vi "WriteJSON.vi"(2 "error in (no error)":errorcluster, 3 "JSONEventInfo":variant) -> (0 "error out":errorcluster, 1 "Boolean":bool)   [LabVIEW 2018]
uses:
  <vilib>/LVH/i3 JSON/JSON Parsing/Get Object Parameter Files/Get Object Parameter - String.vi
  Global Variables.vi
  <vilib>/LVH/i3 JSON/JSON Generation/Create Value Files/Create Value - Object.vi
  <vilib>/LVH/i3 JSON/JSON Generation/Add Object Parameter Files/Add Object Parameter - Object.vi
  <vilib>/LVH/i3 JSON/JSON Generation/Add Object Parameter Files/Add Object Parameter - String.vi
  <vilib>/LVH/i3 JSON/JSON Generation/Append to Array Files/Append to Array - Object.vi
  <vilib>/LVH/i3 JSON/i3-json.lvlib
panel:
  out "JSONpath":path
  in  "String 2":string
  out "concatenated string":string
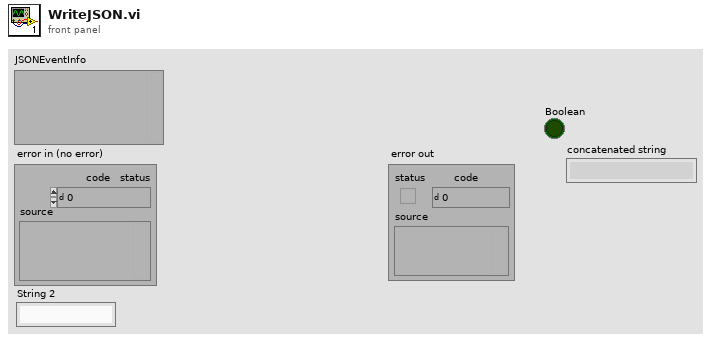
[diagram p1: front panel]
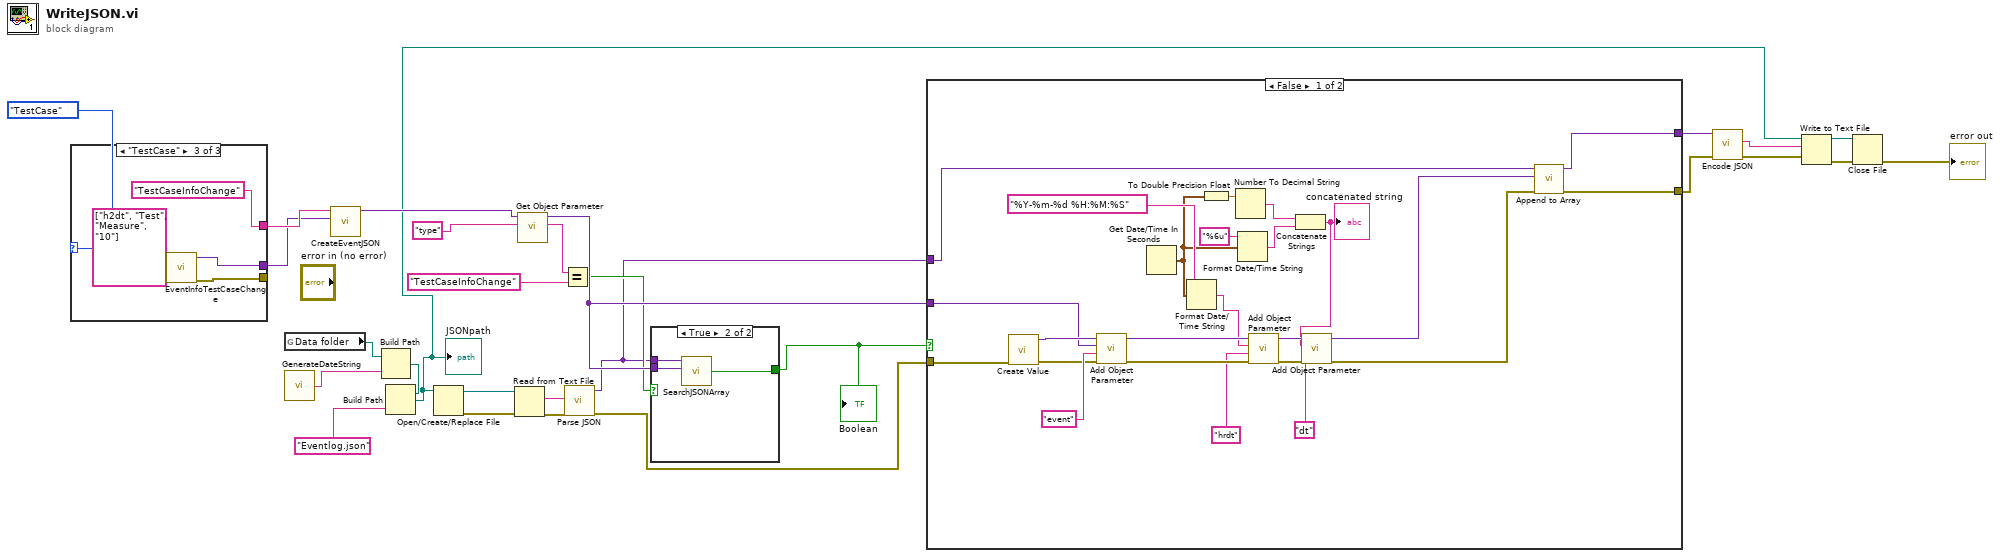
[diagram p0: block diagram]
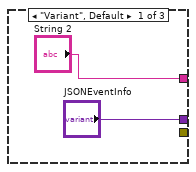
[diagram p3: hidden frame]
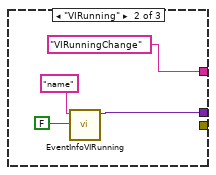
[diagram p4: hidden frame]
diagram:
  n1 = case shown="\"TestCase\"" enum16{"Variant", "TestCase", "VIRunning"}."TestCase" {
    tunnel: ["JSONEventInfo" w34 w38] -> w12
    tunnel: [_ _ w36] -> _
    tunnel: ["String 2" "VIRunningChange" "TestCaseInfoChange"] -> w13
    frame "Variant", Default {
    }
    frame "VIRunning" {
      n2 = call "EventInfoVIRunning.vi"("OnOff"=FALSE, "name"="name") -> ("eventinfoJSON"=w34:variant)  [unwired: 8 in, 1 out]
    }
    frame "TestCase" {
      n3 = call "EventInfoTestCaseChange.vi"("TestCaseInfo"=string[] ["h2dt", "Test", "Measure", "10"]) -> ("error out"=w36:errorcluster, "JSON Tree out (JSON Object)"=w38:variant)  [unwired: 9 in]
    }
  }
  n4 = global read "Global Variables.vi" "Data folder"() -> (w27:path)
  n5 = call "GenerateDateString.vi"() -> ("String"=w28:string)
  n6 = call "CreateEventJSON.vi"("eventinfo"=w12, "type"=w13) -> ("eventJSON"=w14:variant)  [unwired: 8 in, 1 out]
  n7 = Build Path(base path=w27, name or relative path=w28) -> (appended path=w26:path)
  n8 = Build Path(base path=w26, name or relative path="Eventlog.json" ("string")) -> (appended path=w1:path)
  "JSONpath" <- w1
  n9 = Open/Create/Replace File(file path (use dialog)=w1) -> (refnum out=w24:refnum<file>, error out=w21:errorcluster)  [unwired: 5 in, 1 out]
  n10 = Read from Text File(file (use dialog)=w24, error in=w21) -> (text=w22:string, error out=w23:errorcluster)  [unwired: 2 in, 2 out]
  n11 = call-poly <vilib>:"Get Object Parameter.vi"("Parameter Name"="type" ("Default Value if JSON Null"), "JSON Tree In (JSON Object)"=w14) -> ("String Value"=w17:string, "JSON Tree Out Passthrough"=w20:variant)  [unwired: 6 in, 2 out]
  n12 = Equal?(x=w17, y="TestCaseInfoChange") -> (x = y?=w18:bool)
  n13 = call <vilib>:"Parse JSON.vi"("error in (no error)"=w23, "JSON String"=w22) -> ("error out"=w4:errorcluster, "JSON Tree"=w10:variant)  [unwired: 6 in, 2 out]
  n14 = case shown="True" w18 {
    selector: w18 -> [w39 _]
    tunnel: w10 -> [_ w42]
    tunnel: w20 -> [_ w41]
    tunnel: [w39 w40] -> w11
    frame False {
    }
    frame True {
      n15 = call "SearchJSONArray.vi"("eventinfoJSON"=w41, "JSONArray"=w42) -> ("Boolean"=w40:bool)  [unwired: 4 in]
    }
  }
  "Boolean" <- w11
  n16 = case shown="False" w11 {
    tunnel: w20 -> [w49 _]
    tunnel: w10 -> [w47 w68]
    tunnel: [w45 w67] -> w3
    tunnel: [w44 w68] -> w5
    tunnel: w4 -> [w43 w67]
    frame False {
      n17 = call-poly <vilib>:"Create Value.vi"("error in (no error)"=w43) -> ("error out"=w50:errorcluster, "JSON Tree"=w51:variant)  [unwired: 9 in]
      n18 = call-poly <vilib>:"Add Object Parameter.vi"("error in (no error)"=w50, "Name"="event", "JSON Object"=w49, "JSON Tree in (JSON Object)"=w51) -> ("error out"=w65:errorcluster, "JSON Tree out (JSON Object)"=w66:variant)  [unwired: 6 in]
      n19 = Get Date/Time In Seconds() -> (seconds since 1Jan1904=w57:timestamp)
      n20 = Format Date/Time String(time format string (%c)="%Y-%m-%d %H:%M:%S", seconds (now)=w57) -> (date/time string=w61:string)  [unwired: 1 in]
      n21 = To Double Precision Float(number=w57) -> (double precision float=w56:dbl)
      n22 = Number To Decimal String(number=w56) -> (decimal integer string=w58:string)  [unwired: 1 in]
      n23 = Format Date/Time String(time format string (%c)="%6u", seconds (now)=w57) -> (date/time string=w59:string)  [unwired: 1 in]
      n24 = call-poly <vilib>:"Add Object Parameter.vi"("error in (no error)"=w65, "Name"="hrdt", "String"=w61, "JSON Tree in (JSON Object)"=w66) -> ("error out"=w54:errorcluster, "JSON Tree out (JSON Object)"=w55:variant)  [unwired: 6 in]
      n25 = Concatenate Strings(w58, w59) -> (w52:string)
      "concatenated string" <- w52
      n26 = call-poly <vilib>:"Add Object Parameter.vi"("error in (no error)"=w54, "Name"="dt", "String"=w52, "JSON Tree in (JSON Object)"=w55) -> ("error out"=w46:errorcluster, "JSON Tree out (JSON Object)"=w48:variant)  [unwired: 6 in]
      n27 = call-poly <vilib>:"Append to Array.vi"("error in (no error)"=w46, "JSON Object"=w48, "JSON Tree in (JSON Array)"=w47) -> ("error out"=w45:errorcluster, "JSON Tree out (JSON Array)"=w44:variant)  [unwired: 7 in]
    }
    frame True {
    }
  }
  n28 = call <vilib>:"Encode JSON.vi"("error in (no error)"=w3, "JSON Tree"=w5) -> ("error out"=w9:errorcluster, "String"=w6:string)  [unwired: 4 in]
  n29 = Write to Text File(file (use dialog)=w1, text=w6, error in=w9) -> (refnum out=w7:refnum<file>, error out=w8:errorcluster)  [unwired: 1 in, 1 out]
  n30 = Close File(refnum=w7, error in=w8) -> (error out=→"error out":errorcluster)  [unwired: 1 out]
